vi "Enqueue_Mapping_Sensor_Data(SubVI).vi"(9 "LaserScan_msg":T1, 10 "Current_Position_out":T2, 11 "Queue in":refnum<queue>) -> ()   [LabVIEW 2017]
uses:
  Ctl/Current_Position.ctl
  Ctl/Mapping_Sensor_Data.ctl
  ROS/LaserScan.ctl
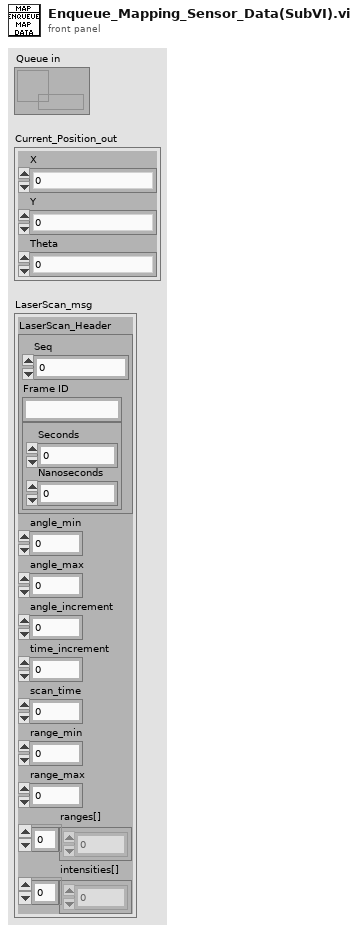
[diagram p1: front panel]
types:
  T1 = typedef "LaserScan.ctl" = cluster{"LaserScan_Header":cluster{"Seq":u32, "Frame ID":string, cluster{"Seconds":i32, "Nanoseconds":i32}}, "angle_min":dbl, "angle_max":dbl, "angle_increment":dbl, "time_increment":dbl, "scan_time":dbl, "range_min":dbl, "range_max":dbl, "ranges[]":dbl[], "intensities[]":dbl[]}
  T2 = typedef "Current_Position.ctl" = cluster{"X":dbl, "Y":dbl, "Theta":dbl}
  T3 = typedef "Mapping_Sensor_Data.ctl" = cluster{"Current_Position":T2, "LaserScan":T1}
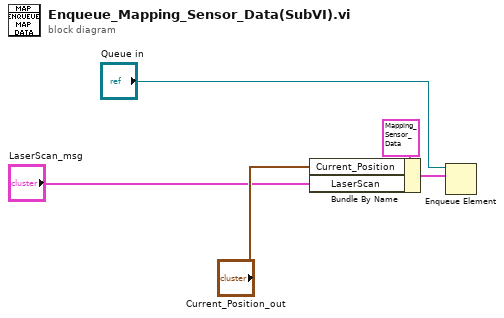
[diagram p0: block diagram]
diagram:
  n1 = Bundle By Name(cluster=T3 {"Current_Position"={"X"=0.0, "Y"=0.0, "Theta"=0.0}, "LaserScan"={"LaserScan_Header"={"Seq"=0, "Frame ID"="", {"Seconds"=0, "Nanoseconds"=0}}, "angle_min"=0.0, "angle_max"=0.0, "angle_increment"=0.0, "time_increment"=0.0, "scan_time"=0.0, "range_min"=0.0, "range_max"=0.0, "ranges[]"=[], "intensities[]"=[]}} ("Cluster"), "Current_Position"="Current_Position_out", "LaserScan"="LaserScan_msg") -> (w4:T3)
  n2 = Enqueue Element(queue="Queue in", element=w4) -> ()  [unwired: 2 in, 3 out]
